vi "getDAQmx.AO_Config.vi"(8 "error in (no error)":errorcluster, 11 "DAQmx.AO in":refnum<class "DAQmx.AO.lvclass">) -> (0 "error out":errorcluster, 2 "output terminal configuration":i32(ring)=-1 items=["Default"=-1, "RSE"=10083, "Differential"=10106, "Pseudodifferential"=12529], 3 "DAQmx.AO out":refnum<class "DAQmx.AO.lvclass">)   [LabVIEW 2016, in "DAQmx.AO.lvclass"]
uses:
  DAQmx.AO.lvclass
  DAQmx.AO.lvclass/DAQmx.AO.ctl
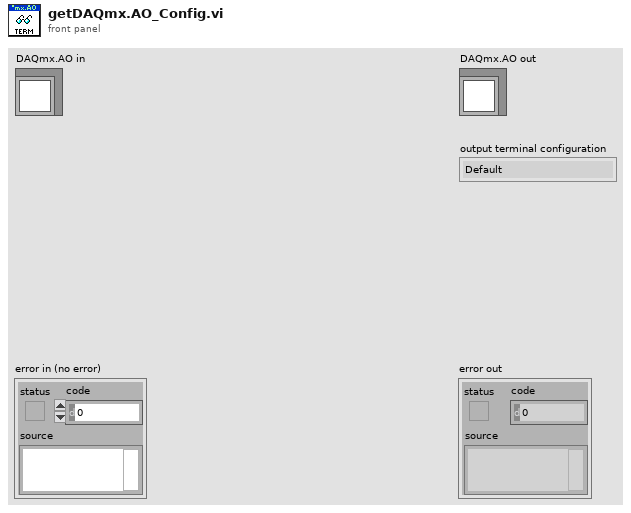
[diagram p1: front panel]
types:
  T1 = typedef "DAQmx.AO.lvclass/AO.Terminal-enum.ctl" = i32
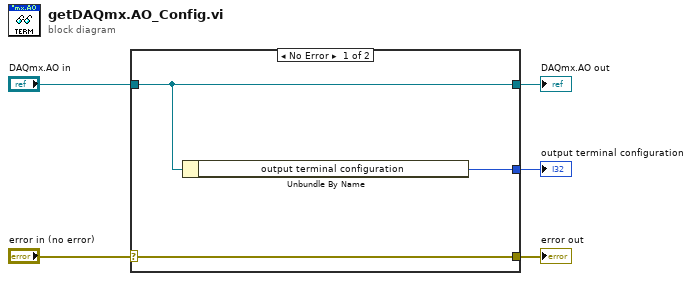
[diagram p0: block diagram]
diagram:
  n1 = case shown="No Error" "error in (no error)" {
    selector: "error in (no error)" -> [w8 w9]
    tunnel: [w8 w9] -> w4
    tunnel: [w7 w10] -> w2
    tunnel: "DAQmx.AO in" -> [w7 w10]
    tunnel: [w6 _] -> w1
    frame No Error {
      n2 = Unbundle By Name(w7) -> ("output terminal configuration"=w6:T1)
    }
    frame Error {
    }
  }
  "error out" <- w4
  "DAQmx.AO out" <- w2
  "output terminal configuration" <- w1
